vi "rs3 Advanced Set Census Enable Reg3.vi"(8 "error in (no error)":errorcluster, 10 "ST_CensusEnableReg":cluster{"uDiameter":u32, "vDiameter":u32}, 11 "device in":u64) -> (0 "error out 2":errorcluster, 1 "error":u64, 3 "Dev out":u64)   [LabVIEW 2017, in "libRealSense3.lvlib"]
doc: "Sets registers inside the ASIC that affect the depth calculations"
uses:
  libRealSense3.lvlib
  realsense2.dll
panel:
  # "RS3 Adv. Set Census Reg"
  # "(C) 2017 Intel Corp.,  AGJ"
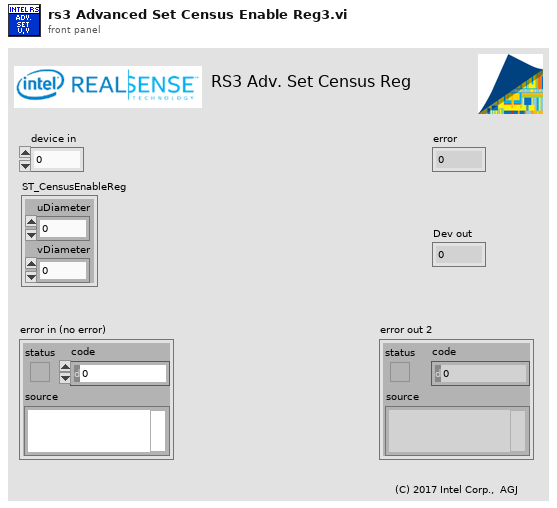
[diagram p1: front panel]
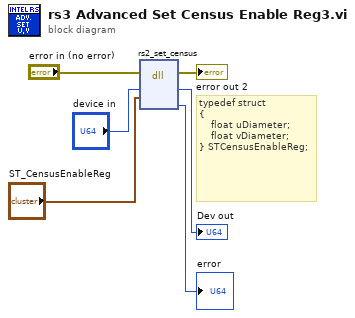
[diagram p0: block diagram]
diagram:
  # "typedef struct\n{\n    float uDiameter;\n    float vDiameter;\n} STCensusEnableReg;"
  n1 = dll-call lib="C:/Users/agrunnet/Documents/libRealSense6/realsense2.dll" fn="rs2_set_census"(error in="error in (no error)", "device"="device in", "ST SLO Threshold"="ST_CensusEnableReg") -> (error out=→"error out 2":errorcluster, "device"=→"Dev out":u64, "error"=→"error":u64)  [unwired: 5 in, 1 out]
